vi "Get_Timestamp.vi"(1 "String":string="%Y%m%d_%H%M%S%3u") -> (0 "date/time string":string)   [LabVIEW 2019]
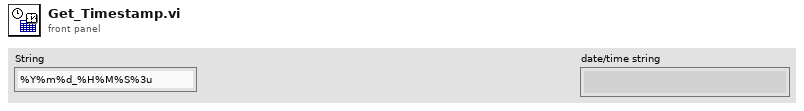
[diagram p1: front panel]
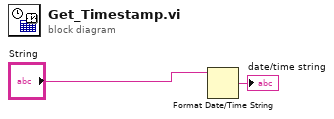
[diagram p0: block diagram]
diagram:
  n1 = Format Date/Time String(time format string (%c)="String") -> (date/time string=→"date/time string":string)  [unwired: 2 in]
